vi "fgt close.vi"(8 "error in (no error)":errorcluster) -> (0 "error out":errorcluster)   [LabVIEW 2016, in "fgt_SDK.lvlib"]
doc: "Close communication with Fluigent instruments and free memory.\nThis function is mandatory, if not called the dll will be automatically closed when exiting your application.\nUsing this function will remove session preferences such as units and limits. If any regulation is running it will stop pressure control."
uses:
  fgt_SDK.lvlib
  dlls/fgt_SDK_32.dll
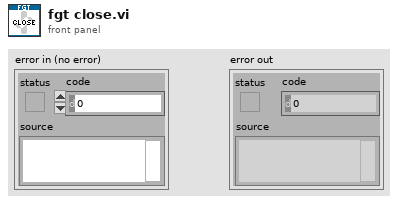
[diagram p1: front panel]
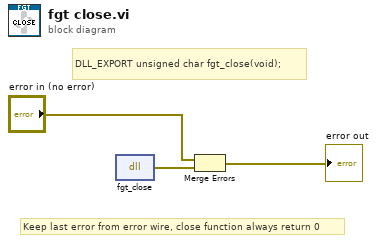
[diagram p0: block diagram]
diagram:
  # "Keep last error from error wire, close function always return 0"
  # "DLL_EXPORT unsigned char fgt_close(void);"
  n1 = dll-call lib="PTH2Zabs D\nMes DocumentsDéveloppementFluigentSDKsfgt-sdk-labviewdllsfgt_SDK_*.*" fn="fgt_close"() -> (error out=w3:errorcluster)  [unwired: 4 in, 1 out]
  n2 = Merge Errors("error in (no error)", w3) -> (→"error out":errorcluster)
